vi "SRV_Start.vi"(0 "Target":enum16{"PC", "SRV", "C Code"}(ring)=enum."SRV") -> (4 "SuperPro":T1)   [LabVIEW 2009]
doc: "Starts a loop that runs N times. N can be specified as a number or a variable (string). You can also define the loop counter (default is i)."
uses:
  <userlib>/SuperPro/OpCodes/_SubVIs/SuperProControl.ctl
panel:
  in  "SuperPro":T1
  # "This LabVIEW item is deprecated.\n\nIt is believed to be unused and will be removed in a future version of SRV."
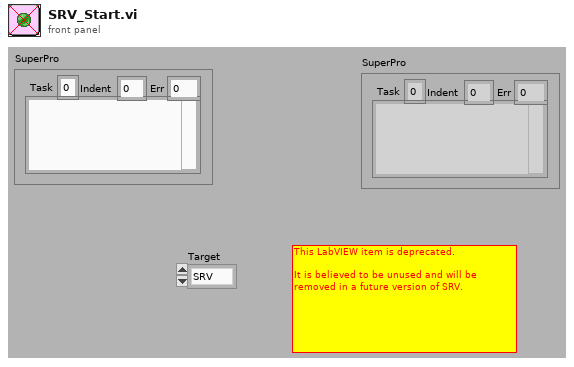
[diagram p1: front panel]
types:
  T1 = typedef "SuperProControl.ctl" = cluster{"Task":i32, "Indent":i32, "Err":i32, "ASM":string}
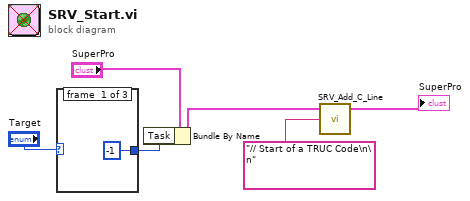
[diagram p0: block diagram]
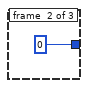
[diagram p2: hidden frame]
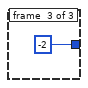
[diagram p3: hidden frame]
diagram:
  n1 = case shown="\"C Code\"" "Target" {
    tunnel: [-1 0 -2] -> w1
    frame #0 {
    }
    frame #1 {
    }
    frame #2 {
    }
  }
  n2 = Bundle By Name(cluster="SuperPro", "Task"=w1) -> (w3:T1)
  n3 = call "SRV_Add_C_Line.vi"("C String"="// Start of a TRUC Code\n\n", "SuperPro in"=w3) -> ("SuperPro out"=→"SuperPro":T1)  [unwired: 3 in]
